vi "8.7-State Updater Test.vi"() -> ()   [LabVIEW 2010]
uses:
  4-High Neurons/4.2/4.2.0 Kalman State.ctl
  <vilib>/Analysis/Matrix/Datatypes/RealMatrix.ctl
  3-Midbrain/3.0 Flow Control/3.0 List of Loops.ctl
  3-Midbrain/3.0-Global.vi
  <vilib>/Analysis/Matrix/Numeric/Conversions/Array To Matrix - RA.vi
  <vilib>/Analysis/baseanly.llb/Real A x B.vi
  <vilib>/Analysis/Matrix/NI_Matrix.lvlib
  <vilib>/Analysis/NI_AALBase.lvlib
panel:
  out "State Update Matrix F":T1
  out "State Vector X":T1
  in  "Stop":bool
  out "State Vector X":T2
  in  "Omega Dot":dbl
  in  "Omega":dbl
  in  "V":dbl
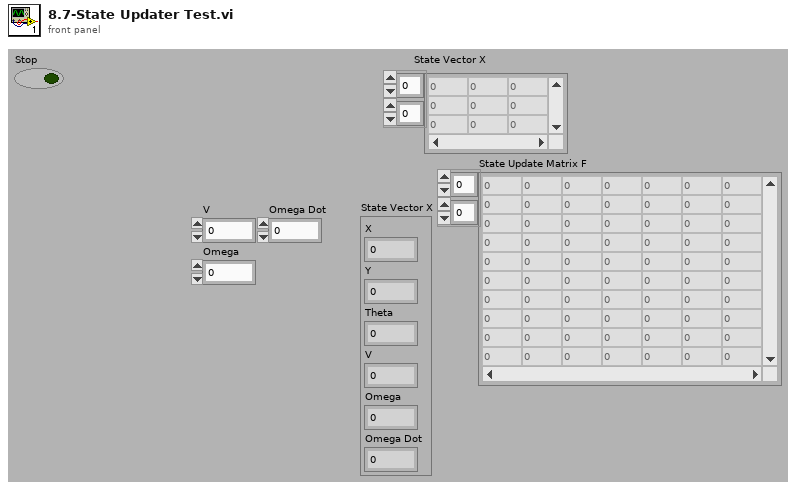
[diagram p1: front panel]
types:
  T1 = typedef "NI_Matrix.lvlib/RealMatrix.ctl" = dbl[][]
  T2 = typedef "4.2.0 Kalman State.ctl" = cluster{"X":dbl, "Y":dbl, "Theta":dbl, "V":dbl, "Omega":dbl, "Omega Dot":dbl}
  T3 = typedef "3.0 List of Loops.ctl" = enum16{"3.0 State Update", "3.0 GUI", "3.1 Act", "3.1 4.7.1 Act UDP", "3.1 Joystick", "3.2 Where", "3.2.0 Kalman Filter", "3.2 4.7.2 Where UDP", "3.3 What", "3.3 4.7.3 What UDP", "3.4 How", "3.4 4.7.4 How UDP", "3.5 Limbic", "3.8 TCP", "3.6 Cerebellum", "3.8 TCP Act"}
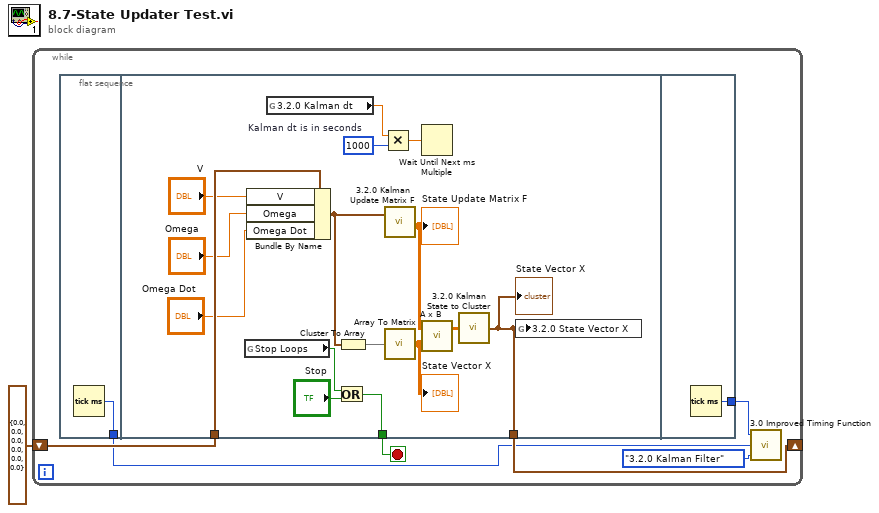
[diagram p0: block diagram]
diagram:
  n1 = while {
    shift-right: [w3] -> _
    shift-left: T2 {"X"=0.0, "Y"=0.0, "Theta"=0.0, "V"=0.0, "Omega"=0.0, "Omega Dot"=0.0} ("State Vector X") -> [w4]
    stop <- w6 stop-if-true
    n2 = flat-sequence {
      tunnel: [w8] -> w2
      tunnel: [w10] -> w6
      tunnel: w4 -> [w23]
      tunnel: [w14] -> w3
      tunnel: [w25] -> w7
      frame #0 {
        n3 = Tick Count (ms)() -> (millisecond timer value=w8:u32)
      }
      frame #1 {
        w16 = 1000  # Kalman dt is in seconds
        n4 = global read "3.0-Global.vi" "Stop Loops"() -> (w24:bool)
        n5 = Bundle By Name(cluster=w23, "V"="V", "Omega"="Omega", "Omega Dot"="Omega Dot") -> (w21:T2)
        n6 = global read "3.0-Global.vi" "3.2.0 Kalman dt"() -> (w17:dbl)
        n7 = Or(x=w24, y="Stop") -> (x .or. y?=w10:bool)
        n8 = Cluster To Array(cluster=w21) -> (array=w22:dbl[])
        n9 = Multiply(x=w17, y=w16) -> (x*y=w15:dbl)
        n10 = call "3.2.0 Kalman Update Matrix F.vi"("State Vector X"=w21) -> ("Update Matrix F"=w20:T1)  [unwired: 4 in]
        "State Update Matrix F" <- w20
        n11 = call-poly <vilib>:"Array To Matrix.vi"("Real 1D Array"=w22) -> ("Real Matrix (Column Vector)"=w19:T1)
        "State Vector X" <- w19
        n12 = Wait Until Next ms Multiple(millisecond multiple=w15) -> ()  [unwired: 1 out]
        n13 = call-poly <vilib>:"A x B.vi"("B"=w19, "A"=w20) -> ("A x B"=w18:T1)  [unwired: 1 out]
        n14 = call "3.2.0 Kalman State to Cluster.vi"("State Variable X 3"=w18) -> ("State Vector X"=w14:T2)
        "State Vector X" <- w14
        n15 = global write "3.0-Global.vi" "3.2.0 State Vector X"(w14) -> ()
      }
      frame #2 {
        n16 = Tick Count (ms)() -> (millisecond timer value=w25:u32)
      }
    }
    n17 = call "3.0 Improved Timing Function.vi"("Loop"=3.0_List_of_Loops."3.2.0 Kalman Filter", "Start"=w2, "End"=w7) -> ()  [unwired: 1 in]
  }
